vi "VolumeSubvi.vi"(1 "Array":dbl[](array[numeric])) -> (0 "Total volume Vd":dbl[](array[numeric]))   [LabVIEW 2021]
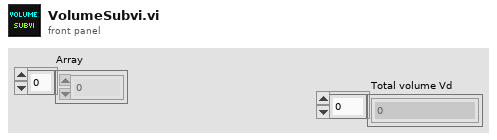
[diagram p1: front panel]
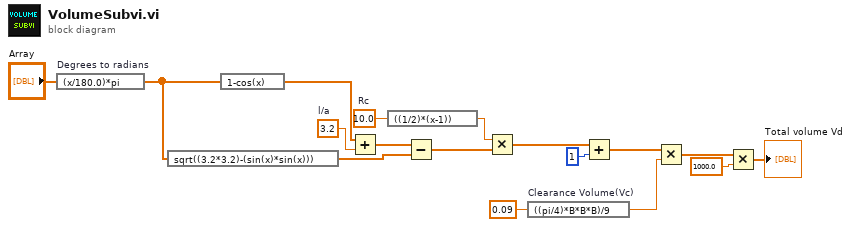
[diagram p0: block diagram]
diagram:
  w10 = 10.0  # Rc
  w15 = 3.2  # l/a
  n1 = expression code="(x/180.0)*pi" "Degrees to radians"("Array") -> (w17:dbl[])
  n2 = expression code="sqrt((3.2*3.2)-(sin(x)*sin(x)))" ("Degrees to radians")(w17) -> (w13:dbl[])
  n3 = expression code="1-cos(x)" ("Degrees to radians")(w17) -> (w16:dbl[])
  n4 = Add(x=w16, y=w15) -> (x+y=w14:dbl[])
  n5 = expression code="((1/2)*(x-1))" ("Degrees to radians")(w10) -> (w11:dbl)
  n6 = Subtract(x=w14, y=w13) -> (x-y=w12:dbl[])
  n7 = Multiply(x=w11, y=w12) -> (x*y=w9:dbl[])
  n8 = expression code="((pi/4)*B*B*B)/9" "Clearance Volume(Vc)"(0.09) -> (w5:dbl)
  n9 = Add(x=w9, y=1 ("Rc")) -> (x+y=w6:dbl[])
  n10 = Multiply(x=w6, y=w5) -> (x*y=w3:dbl[])
  n11 = Multiply(x=w3, y=1000.0) -> (x*y=→"Total volume Vd":dbl[])
